vi "Interpolate 2D (1d xi,yi).vi"(4 "ntimes":i32=1, 6 "yi":dbl[](array[numeric]), 7 "method":i32(ring) items=["nearest", "bilinear", "bicubic", "bicubic spline"], 8 "xi":dbl[](array[numeric]), 9 "Y":dbl[](array[numeric]), 10 "X":dbl[](array[numeric]), 11 "Z":dbl[][](array[numeric])) -> (0 "error":i32, 1 "yi used":dbl[][](array[numeric]), 2 "xi used":dbl[][](array[numeric]), 3 "zi":dbl[][](array[numeric]))   [LabVIEW 2017, in "NI_Gmath.lvlib"]
doc: "Performs two-dimensional interpolation using a selected interpolation method based on the lookup table defined by <B>X</B>, <B>Y</B>, and <B>Z</B>, where <B>Z</B> is a 2D array. You must manually select the polymorphic instance to use."
uses:
  NI_Gmath.lvlib
panel:
  # "Interpolate 2D (1d xi,yi)"
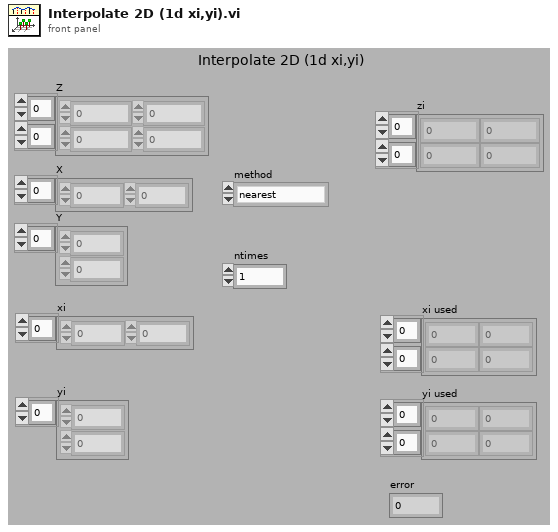
[diagram p1: front panel]
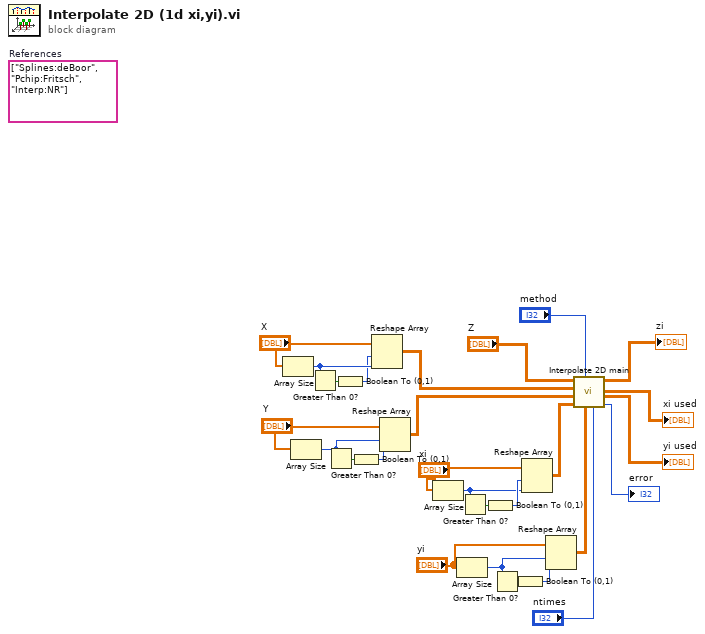
[diagram p0: block diagram]
diagram:
  (unwired) string[] ["Splines:deBoor", "Pchip:Fritsch", "Interp:NR"]  # References
  n1 = Array Size(array="X") -> (size(s)=w19:i32)
  n2 = Array Size(array="Y") -> (size(s)=w13:i32)
  n3 = Greater Than 0?(x=w19) -> (x > 0?=w16:bool)
  n4 = Greater Than 0?(x=w13) -> (x > 0?=w7:bool)
  n5 = Boolean To (0,1)(Boolean=w16) -> (0, 1=w18:i16)
  n6 = Boolean To (0,1)(Boolean=w7) -> (0, 1=w14:i16)
  n7 = Reshape Array("X", w18, w19) -> (w17:dbl[][])
  n8 = Reshape Array("Y", w13, w14) -> (w12:dbl[][])
  n9 = Array Size(array="xi") -> (size(s)=w4:i32)
  n10 = Array Size(array="yi") -> (size(s)=w11:i32)
  n11 = Greater Than 0?(x=w4) -> (x > 0?=w6:bool)
  n12 = Boolean To (0,1)(Boolean=w6) -> (0, 1=w5:i16)
  n13 = Greater Than 0?(x=w11) -> (x > 0?=w9:bool)
  n14 = Boolean To (0,1)(Boolean=w9) -> (0, 1=w10:i16)
  n15 = Reshape Array("xi", w5, w4) -> (w2:dbl[][])
  n16 = Reshape Array("yi", w11, w10) -> (w1:dbl[][])
  n17 = call "Interpolate 2D main.vi"("ntimes"="ntimes", "yi"=w1, "method"="method", "xi"=w2, "Y"=w12, "X"=w17, "Z"="Z") -> ("error"=→"error":i32, "yi used"=→"yi used":dbl[][], "xi used"=→"xi used":dbl[][], "zi"=→"zi":dbl[][])  [unwired: 1 in]
